vi "LINX - Ultrasonic.vi"() -> ()   [LabVIEW 2011, in "LVH-LINX.lvlib"]
doc: "Measure distance using an ultrasonic range finder."
uses:
  vi.lib/LabVIEW Hacker/LINX/LVH-LINX.lvlib
  vi.lib/LabVIEW Hacker/LINX/Public/Sensors/Ultrasonic/Ultrasonic.lvlib
panel:
  out "Distance (cm)":dbl(slide) scale=0.0..100.0
  in  "Digital Input Channel":u8
  in  "Serial Port":refnum<visa-resource-name>
  out "Loop Rate (Hz)":u32
  in  "Stop Button":bool
  # "Ultrasonic Example\n\nThis example demonstrates how to measure distance using an ultrasonic sensor.\n\nInstructions\n1. Select the COM Port associated with the LINX Device.\n2. Select the Digital Input channel connected to the ultrasonic sensor.\n3. Click the Run Arrow."
  # "Circuit Schematic"
  # "LINX Device Settings"
  # "Distance (cm)"
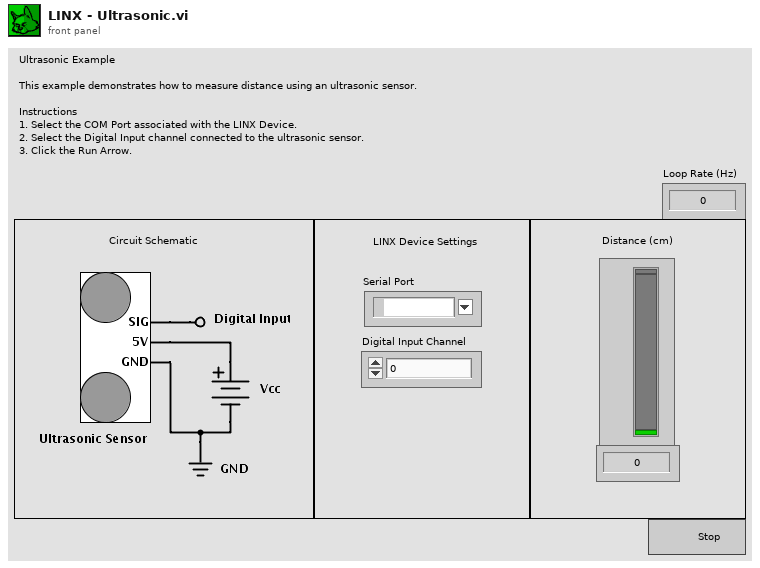
[diagram p1: front panel]
types:
  T1 = typedef "LVH-LINX.lvlib/LINX Ref.ctl" = cluster{"Platform":T2, "Interface":T3, "LINX Device Config":T4}
  T2 = typedef "LVH-LINX.lvlib/Platform.ctl" = enum16{"LINX", "myRIO"}
  T3 = typedef "LVH-LINX.lvlib/Interface.ctl" = enum16{"Serial", "TCP"}
  T4 = typedef "LVH-LINX.lvlib/Device.lvlib/LINX Device Config.ctl" = cluster{"Interface":T3, "COM Port":refnum<visa-resource-name>, "TCP Configuration":T5, "Device Family":T6, "Device ID":u8, "Device Name":string, "TCP Ref":refnum<k5>}
  T5 = typedef "LVH-LINX.lvlib/Device.lvlib/TCP Config.ctl" = cluster{"IP Address":string, "Port":u16}
  T6 = typedef "LVH-LINX.lvlib/Device Family.ctl" = enum8{"National Instruments", "Digilent", "Arduino"}
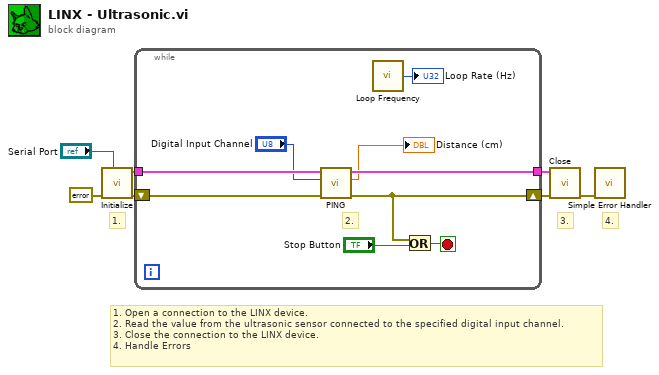
[diagram p0: block diagram]
diagram:
  # "1. Open a connection to the LINX device.\n2. Read the value from the ultrasonic sensor connected to the specified digital input channel.\n3. Close the connection to the LINX device.\n4. Handle Errors"
  # "4."
  # "3."
  # "1."
  n1 = call "Initialize.vi"("Serial Port"="Serial Port", "Error In"=errorcluster {"status"=FALSE, "code"=0, "source"=""}) -> ("Error Out"=w6:errorcluster, "LINX Ref"=w7:T1)  [unwired: 7 in, 1 out]
  n2 = while {
    tunnel: w7 -> [w13]
    tunnel: [w12] -> w5
    shift-right: [w11] -> w4
    shift-left: w6 -> [w9]
    stop <- w16 stop-if-true
    # "2."
    n3 = call "PING.vi"("Error In"=w9, "SIG Pin (DIO)"="Digital Input Channel", "LINX Resource"=w13) -> ("Error Out"=w11:errorcluster, "Centimeters"=→"Distance (cm)":dbl, "LINX Resource"=w12:T1)  [unwired: 5 in, 1 out]
    n4 = call "Loop Frequency.vi"() -> ("Loop Rate (Hz)"=→"Loop Rate (Hz)":u32)
    n5 = Or(x=w11, y="Stop Button") -> (x .or. y?=w16:bool)
  }
  n6 = call "Close.vi"("Error In"=w4, "LINX Resource"=w5) -> ("Error Out"=w2:errorcluster)  [unwired: 8 in, 1 out]
  n7 = call <vilib>:"Simple Error Handler.vi"("error in (no error)"=w2) -> ()  [unwired: 4 in, 5 out]
